vi "FPGA Main (David Documentation).vi"() -> ()   [LabVIEW 2015]
uses:
  Sub VIs/Utilities/Start Boolean.ctl
  <vilib>/Platform/TimedLoop/XDataNode/timing_clust.ctl
  <vilib>/Platform/TimedLoop/XDataNode/nitl_modes.ctl
  <vilib>/Platform/TimedLoop/XDataNode/wakeup.ctl
  <vilib>/rvi/Emulation/niFpgaSctlEmulationGetInTimedLoop.vi
  <vilib>/rvi/Emulation/niFpgaEmulationReportErrorSimple.vi
  <vilib>/rvi/Emulation/niFpgaGetClockAttributes.vi
  <vilib>/rvi/Emulation/niFpgaCriticalErrorInLSC.vi
  <vilib>/rvi/eio/common/nirviEmuTemplateMethod_errors.vi
  <vilib>/Platform/TimedLoop/XDataNode/XDataNode.xnode
  <vilib>/eio/EIONode/EIONode.xnode
  <vilib>/Platform/TimedLoop/XDataNode/XDNodeRunTimeDep.lvlib
panel:
  in  "I2S.BitCount":u16=32
  in  "I2S.MUTEN":bool
  out "I2S.DataChannel":bool
  in  "I2S.WordLength":u16=32
  in  "I2C.Configuration":u8
  out "I2C.Status":u8
  out "I2C.DataIn":u8
  in  "I2C.Counter":u16=187
  in  "I2C.Address":u8
  in  "I2C.Control":u8
  in  "I2C.GO":T1
  in  "I2C.DataOut":u8
  # "Overview: This VI is run on FPGA target, implemented I2C protocol and I2S protocol.\nRequirements: LabVIEW FPGA Module, Xilinx Compilation Tools for Vivado, LabVIEW Support for Digital Systems Development Board\nInstructions: See the details from instructions section on front panel of Desktop Main.vi."
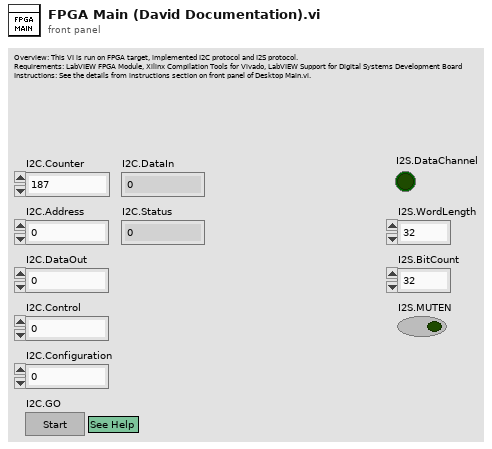
[diagram p1: front panel]
types:
  T1 = typedef "Start Boolean.ctl" = bool
  T2 = typedef "XDNodeRunTimeDep.lvlib/timing_clust.ctl" = cluster{"Expected End [f-1]":u64, "Actual End [f-1]":u64, "Finished Late? [f-1]":bool, "Expected End [i-1]":u64, "Actual End [i-1]":u64, "Finished Late? [i-1]":bool, "Expected Start [i]":u64, "Actual Start [i]":u64, "Expected Start [f]":u64, "Actual Start [f]":u64, "Source Name":string, "Structure Name":string, "Period":i64, "Deadline":i64, "Offset":i64, "Start":i64, "Priority":i32, "Timeout":i32, "Mode":T3, "Wakeup Reason":T4, "Error":errorcluster, "Source Type":string, "Secondary Source Type":string, "Global End Time":u64, "Global Start Time":u64, "Frame Duration":u64, "Iteration Duration":u64, "Assigned CPU":i32, "I/O Scan Engine Mode":u32}
  T3 = typedef "XDNodeRunTimeDep.lvlib/nitl_modes.ctl" = enum32{"No Change", "Process missed periods, maintain original phase", "Discard missed periods, maintain original phase", "Process missed periods, ignore original phase", "Discard missed periods, ignore original phase"}
  T4 = typedef "XDNodeRunTimeDep.lvlib/wakeup.ctl" = enum32{"Normal", "Aborted", "Asynchronous wakeup", "Timing source error", "Timed loop error", "Timeout"}
  T5 = typedef "Audio Signals.ctl" = cluster{"Left Data":u32, "Right Data":u32}
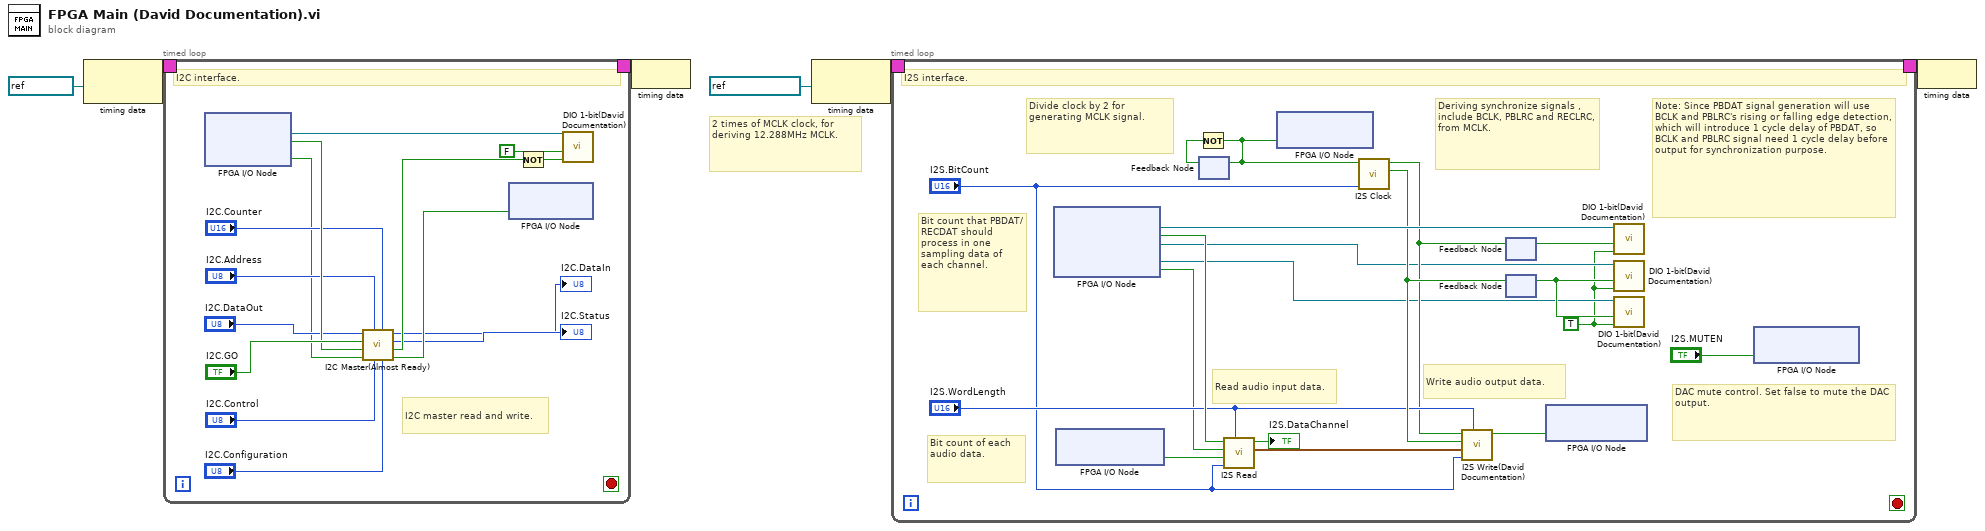
[diagram p0: block diagram]
diagram:
  # "2 times of MCLK clock, for deriving 12.288MHz MCLK."
  n1 = node-c288(refnum<k21> "40MHz" ("Source Name")) -> (w6:T2)
  n2 = timed-loop {
    timing: w6 -> [_]
    timing-out: [_] -> w5
    stop <- _ stop-if-true
    # "I2C master read and write."
    # "I2C interface."
    n3 = xnode "FPGA I/O Node"() -> ("AC_SDA"=w16:bool, "FPGA I/O Out"=w17:refnum<k21>, "AC_SCL"=w7:bool)  [unwired: 2 in, 1 out]
    n4 = call "I2C Master(Almost Ready).vi"("Configuration"="I2C.Configuration", "Counter"="I2C.Counter", "Control"="I2C.Control", "Address In"="I2C.Address", "SCL_IN"=w7, "SDA_IN"=w16, "Execute?"="I2C.GO", "Data Out"="I2C.DataOut") -> ("SCL_OUT"=w15:bool, "SDA_OUT"=w19:bool, "Status"=→"I2C.Status":u8, "Data In"=→"I2C.DataIn":u8)
    n5 = xnode "FPGA I/O Node"("AC_SCL"=w15) -> ()  [unwired: 1 in, 1 out]
    n6 = Not(x=w19) -> (.not. x?=w20:bool)
    n7 = call "DIO 1-bit(David Documentation).vi"("DIR"=w20, "OUT"=FALSE, "DIO Refnum"=w17) -> ()  [unwired: 8 in, 1 out]
  }
  n8 = node-c288(w5) -> ()
  n9 = node-c288(refnum<k21> "24.58MHz" ("Source Name")) -> (w4:T2)
  n10 = timed-loop {
    timing: w4 -> [_]
    timing-out: [_] -> w3
    stop <- _ stop-if-true
    w24 = TRUE ("DIR")
    # "Note: Since PBDAT signal generation will use BCLK and PBLRC's rising or falling edge detection, which will introduce 1 cycle delay of PBDAT, so BCLK and PBLRC signal need 1 cycle delay before output for synchronization purpose."
    # "Write audio output data."
    # "Bit count of each audio data."
    # "Bit count that PBDAT/RECDAT should process in one sampling data of each channel."
    # "Read audio input data."
    # "Deriving synchronize signals , include BCLK, PBLRC and RECLRC, from MCLK."
    # "Divide clock by 2 for generating MCLK signal."
    # "DAC mute control. Set false to mute the DAC output."
    # "I2S interface."
    n11 = xnode "FPGA I/O Node"() -> ("AC_BCLK"=w37:bool, "FPGA I/O Out"=w42:refnum<k21>, "FPGA I/O Out"=w32:refnum<k21>, "AC_RECLRC"=w30:bool, "FPGA I/O Out"=w31:refnum<k21>)  [unwired: 3 in, 1 out]
    n12 = xnode "FPGA I/O Node"() -> ("AC_RECDAT"=w40:bool)  [unwired: 1 in, 1 out]
    n13 = feedback #1() -> (w39:bool)  [unwired: 1 in]
    n14 = Not(x=w39) -> (.not. x?=w26:bool)
    n15 = feedback-in #1(w26) -> ()
    n16 = call "I2S Read.vi"("I2S.WL"="I2S.WordLength", "I2S.BitCount"="I2S.BitCount", "I2S.RECDAT IN"=w40, "I2S.RECLRC IN"=w30, "I2S.BCLK IN"=w37) -> ("Audio Signals"=w28:T5, "Data Channel"=→"I2S.DataChannel":bool)  [unwired: 5 in]
    n17 = xnode "FPGA I/O Node"("AC_MCLK"=w26) -> ()  [unwired: 1 in, 1 out]
    n18 = call "I2S Clock.vi"("I2S.BitCount"="I2S.BitCount", "I2S.MCLK"=w26) -> ("I2S.PBLRC/RECLRC OUT"=w36:bool, "I2S.BCLK OUT"=w33:bool)  [unwired: 8 in]
    n19 = call "I2S Write(David Documentation).vi"("I2S.WL"="I2S.WordLength", "I2S.BitCount"="I2S.BitCount", "Audio Signals"=w28, "I2S.PBLRC"=w36, "I2S.BCLK IN"=w33) -> ("I2S.PBDAT OUT"=w25:bool)  [unwired: 6 in]
    n20 = feedback-in #2(w33) -> ()
    n21 = feedback #2() -> (w34:bool)  [unwired: 1 in]
    n22 = feedback-in #3(w36) -> ()
    n23 = feedback #3() -> (w38:bool)  [unwired: 1 in]
    n24 = xnode "FPGA I/O Node"("AC_PBDAT"=w25) -> ()  [unwired: 1 in, 1 out]
    n25 = call "DIO 1-bit(David Documentation).vi"("DIR"=w24, "OUT"=w34, "DIO Refnum"=w42) -> ()  [unwired: 8 in, 1 out]
    n26 = call "DIO 1-bit(David Documentation).vi"("DIR"=w24, "OUT"=w38, "DIO Refnum"=w32) -> ()  [unwired: 8 in, 1 out]
    n27 = call "DIO 1-bit(David Documentation).vi"("DIR"=w24, "OUT"=w38, "DIO Refnum"=w31) -> ()  [unwired: 8 in, 1 out]
    n28 = xnode "FPGA I/O Node"("AC_MUTEN"="I2S.MUTEN") -> ()  [unwired: 1 in, 1 out]
  }
  n29 = node-c288(w3) -> ()
